vi "Get Latest NIVS Version for Year.vi"(8 "error in (no error)":errorcluster, 10 "software components":T1[](array[typedef]) caption="available software components" {"component type" items=["standard", "hidden", "system", "unknown", "startup"]}) -> (0 "error out":errorcluster, 1 "found":bool, 2 "nivs software to install":T1[](array[typedef]) {"component type" items=["standard", "hidden", "system", "unknown", "startup", "image"]})   [LabVIEW 2013]
uses:
  <vilib>/nisyscfg/Software 1.2.ctl
  <vilib>/nisyscfg/Component Type.ctl
  <vilib>/nisyscfg/nisyscfg.lvlib
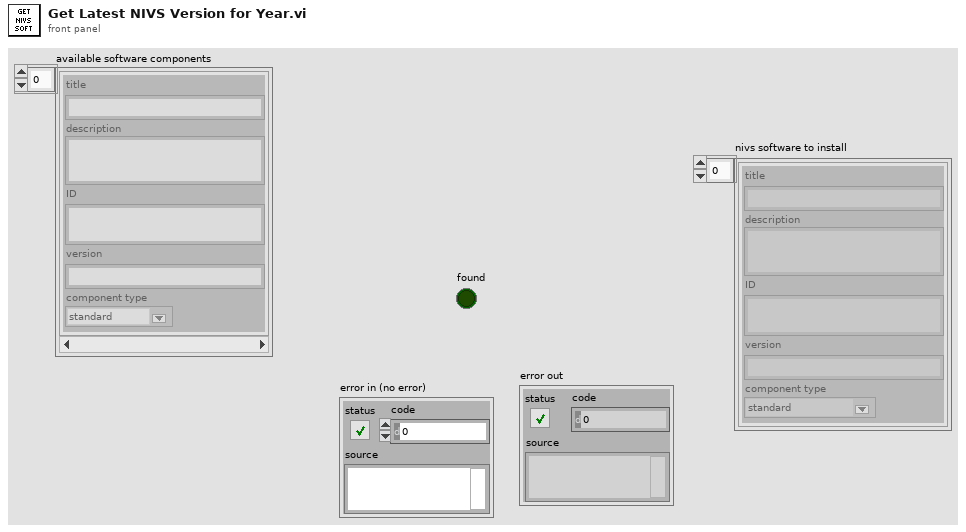
[diagram p1: front panel]
types:
  T1 = typedef "nisyscfg.lvlib/Software 1.2.ctl" = cluster{"title":string, "description":string, "ID":string, "version":string, "component type":T2}
  T2 = typedef "nisyscfg.lvlib/Component Type.ctl" = u32
  T3 = cluster{cluster{i32, i32, i32, i32}, "Software":T1}
  T4 = cluster{cluster{i32, i32, i32, i32}, "Software":T1}[]
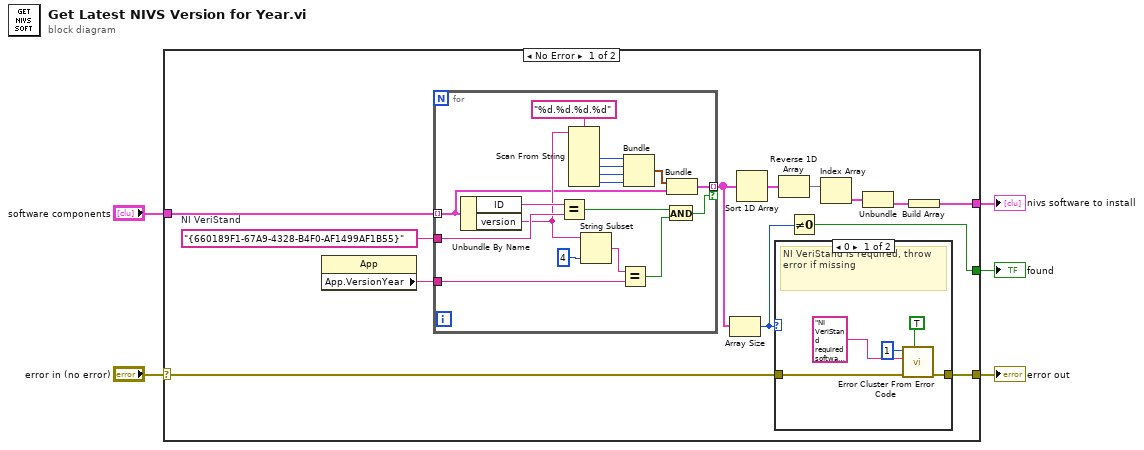
[diagram p0: block diagram]
diagram:
  n1 = case shown="No Error" "error in (no error)" {
    selector: "error in (no error)" -> [w9 w42]
    tunnel: [w8 _] -> w2
    tunnel: "software components" -> [w12 _]
    tunnel: [w10 w42] -> w3
    tunnel: [w6 _] -> w1
    frame No Error {
      w18 = "{660189F1-67A9-4328-B4F0-AF1499AF1B55}"  # NI VeriStand
      n2 = property class="App"() -> ("App.VersionYear"=w17:string)  [unwired: 2 in, 2 out]
      n3 = for {
        tunnel: w12 -> [w27] mode=indexing
        tunnel: w18 -> [w40]
        tunnel: w17 -> [w36]
        tunnel: [w26] -> w11 mode=indexing if=w25
        n4 = Unbundle By Name(w27) -> ("ID"=w41:string, "version"=w29:string)
        n5 = Equal?(x=w41, y=w40) -> (x = y?=w39:bool)
        n6 = Scan From String(format string="%d.%d.%d.%d", input string=w29) -> (output 1=w31:i32, output 2=w34:i32, output 3=w33:i32, output 4=w32:i32)  [unwired: 6 in, 3 out]
        n7 = String Subset(string=w29, length (rest)=4 ("length (rest)")) -> (substring=w37:string)  [unwired: 1 in]
        n8 = Equal?(x=w37, y=w36) -> (x = y?=w35:bool)
        n9 = Bundle(w31, w34, w33, w32) -> (w28:cluster{i32, i32, i32, i32})  [unwired: 1 in]
        n10 = And(x=w39, y=w35) -> (x .and. y?=w25:bool)
        n11 = Bundle(w28, "Software"=w27) -> (w26:T3)  [unwired: 1 in]
      }
      n12 = Array Size(array=w11) -> (size(s)=w7:i32)
      n13 = Sort 1D Array(array=w11) -> (sorted array=w16:T4)
      n14 = case shown="0" w7 {
        tunnel: [w23 w24] -> w10
        tunnel: w9 -> [w22 w24]
        frame 0 {
          # "NI VeriStand is required, throw error if missing"
          n15 = call <vilib>:"Error Cluster From Error Code.vi"("show call chain? (False)"=TRUE, "error in (no error)"=w22, "error message (\"\")"="NI VeriStand required software missing. Reinstall NI VeriStand." ("error message (\"\")"), "error code (0)"=1) -> ("error out"=w23:errorcluster)  [unwired: 5 in]
        }
        frame Default {
        }
      }
      n16 = Reverse 1D Array(array=w16) -> (reversed array=w15:T4)
      n17 = Not Equal To 0?(x=w7) -> (x != 0?=w6:bool)
      n18 = Index Array(array=w15) -> (element=w14:T3)  [unwired: 1 in]
      n19 = Unbundle(w14) -> ("Software"=w13:T1)  [unwired: 1 out]
      n20 = Build Array(w13) -> (w8:T1[])
    }
    frame Error {
    }
  }
  "error out" <- w3
  "nivs software to install" <- w2
  "found" <- w1
